vi "Data Message Type.vi"(10 "Group Data Type":T1) -> (2 "Message Type":string)   [LabVIEW 2020, in "Vecto.lvlib" / "RemoteDataService.lvclass"]
uses:
  RemoteDataService.lvclass
  RemoteDataService.lvclass/RemoteDataService.ctl
  Group Data Type.ctl
  VectoConfig/VectoConfig.lvlib
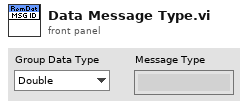
[diagram p1: front panel]
types:
  T1 = typedef "VectoConfig.lvlib/Group Data Type.ctl" = enum16{"Double", "String", "Bool"}
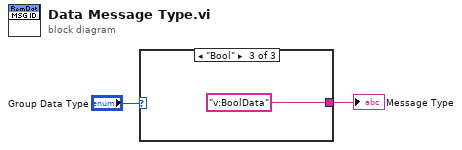
[diagram p0: block diagram]
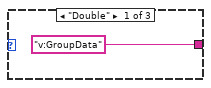
[diagram p2: hidden frame]
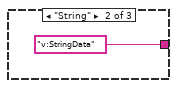
[diagram p3: hidden frame]
diagram:
  n1 = case shown="\"Bool\"" "Group Data Type" {
    tunnel: ["v:GroupData" ("type") "v:StringData" ("type") "v:BoolData" ("type")] -> w1
    frame "Double" {
    }
    frame "String" {
    }
    frame "Bool" {
    }
  }
  "Message Type" <- w1
